vi "Read Y.vi"(8 "error in (no error)":errorcluster, 11 "Y (1Ch) in":refnum<class "Y (1 Ch).lvclass">) -> (0 "error out":errorcluster, 2 "Y":dbl[](array[numeric]), 3 "Y (1Ch) out":refnum<class "Y (1 Ch).lvclass">)   [LabVIEW 2017, in "Y (1 Ch).lvclass"]
uses:
  <vilib>/addons/_NISVFA/_Shared subVIs/Data Objects/Y (DBL)/Y (1 Ch).lvclass
  <vilib>/addons/_NISVFA/_Shared subVIs/Data Objects/Y (DBL)/Y (1 Ch).lvclass/Y (1 Ch).ctl
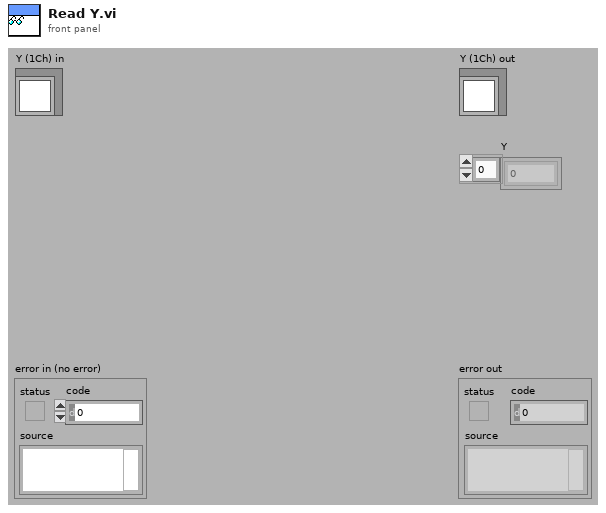
[diagram p1: front panel]
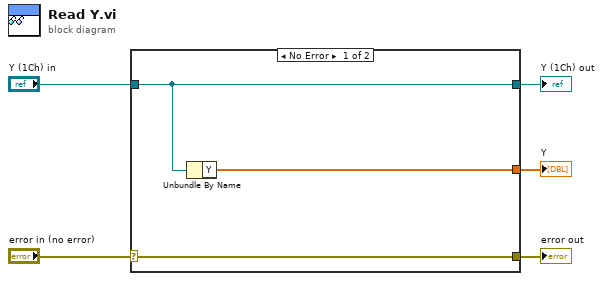
[diagram p0: block diagram]
diagram:
  n1 = case shown="No Error" "error in (no error)" {
    selector: "error in (no error)" -> [w8 w9]
    tunnel: [w8 w9] -> w4
    tunnel: [w7 w10] -> w2
    tunnel: "Y (1Ch) in" -> [w7 w10]
    tunnel: [w6 _] -> w1
    frame No Error {
      n2 = Unbundle By Name(w7) -> ("Y"=w6:dbl[])
    }
    frame Error {
    }
  }
  "error out" <- w4
  "Y (1Ch) out" <- w2
  "Y" <- w1
